vi "Votes Cast Count.vi"(11 "map":map{i32, T1}(c390)) -> (3 "Vote Count":i32)   [LabVIEW 2019]
uses:
  SubVIs/Voter Info.ctl
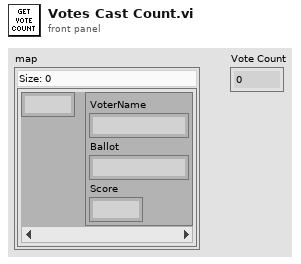
[diagram p1: front panel]
types:
  T1 = typedef "Voter Info.ctl" = cluster{"VoterName":string, "Ballot":string, "Score":i32}
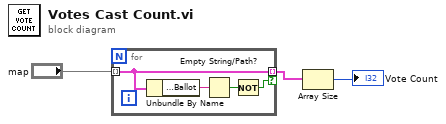
[diagram p0: block diagram]
diagram:
  n1 = for {
    tunnel: "map" -> [w7] mode=indexing
    tunnel: [w7] -> w2 mode=indexing if=w4
    n2 = Unbundle By Name(w7) -> ("VoterInfo.Ballot"=w6:string)
    n3 = Empty String/Path?(string/path=w6) -> (empty?=w5:bool)
    n4 = Not(x=w5) -> (.not. x?=w4:bool)
  }
  n5 = Array Size(array=w2) -> (size(s)=→"Vote Count":i32)
